vi "simple_test.vi"(8 "error in (no error)":errorcluster) -> ()   [LabVIEW 2020]
uses:
  Doc/Doc.lvclass
  Table/Table.lvclass
  Item/Item.lvclass
  Value/Value.lvclass
panel:
  out "integer_value":i64
  out "toml_string":string
  out "tables":string[](array[string])
  out "error out":errorcluster
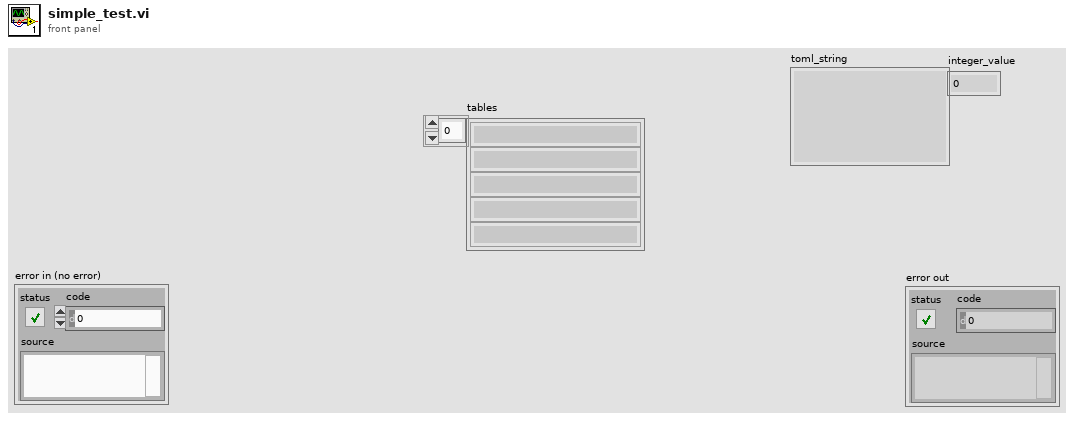
[diagram p1: front panel]
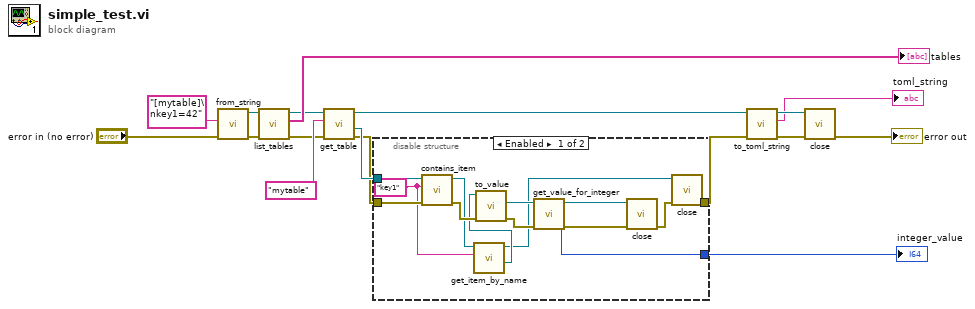
[diagram p0: block diagram]
diagram:
  n1 = call "from_string.vi"("error in (no error)"="error in (no error)", "toml"="[mytable]\nkey1=42") -> ("error out"=w14:errorcluster, "Doc out"=w15:refnum<class "Doc.lvclass">)  [unwired: 8 in]
  n2 = call "list_tables.vi"("error in (no error)"=w14, "Doc in"=w15) -> ("error out"=w5:errorcluster, "table_names"=→"tables":string[], "Doc out"=w8:refnum<class "Doc.lvclass">)  [unwired: 7 in]
  n3 = call "get_table.vi"("error in (no error)"=w5, "table_name"="mytable", "Doc in"=w8) -> ("error out"=w3:errorcluster, "Table"=w4:refnum<class "Table.lvclass">, "Doc out"=w6:refnum<class "Doc.lvclass">)  [unwired: 6 in]
  n4 = disable-structure shown="Enabled" {
    disable-tunnel: w4 -> [w31 _]
    disable-tunnel: w3 -> [w30 _]
    disable-tunnel: [w26 _] -> w2
    disable-tunnel: [w22 _] -> w1
    frame Enabled {
      w21 = "key1" ("item_name")
      n5 = call "contains_item.vi"("error in (no error)"=w30, "item_name"=w21, "Table in"=w31) -> ("error out"=w28:errorcluster, "Table out"=w19:refnum<class "Table.lvclass">)  [unwired: 6 in, 1 out]
      n6 = call "get_item_by_name.vi"("item_name"=w21, "Table in"=w19) -> ("Item"=w20:refnum<class "Item.lvclass">, "Table out"=w18:refnum<class "Table.lvclass">)  [unwired: 7 in, 1 out]
      n7 = call "to_value.vi"("error in (no error)"=w28, "Item in"=w20) -> ("error out"=w27:errorcluster, "Value out"=w29:refnum<class "Value.lvclass">)  [unwired: 8 in]
      n8 = call "get_value_for_integer.vi"("error in (no error)"=w27, "Value in"=w29) -> ("error out"=w24:errorcluster, "integer_value"=w26:i64, "Value out"=w25:refnum<class "Value.lvclass">)  [unwired: 7 in]
      n9 = call "close.vi"("error in (no error)"=w24, "Value in"=w25) -> ("error out"=w23:errorcluster)  [unwired: 9 in]
      n10 = call "close.vi"("error in (no error)"=w23, "Table in"=w18) -> ("error out"=w22:errorcluster)  [unwired: 9 in]
    }
    frame Disabled {
    }
  }
  "integer_value" <- w2
  n11 = call "to_toml_string.vi"("error in (no error)"=w1, "Doc in"=w6) -> ("error out"=w12:errorcluster, "toml_string"=→"toml_string":string, "Doc out"=w11:refnum<class "Doc.lvclass">)  [unwired: 7 in]
  n12 = call "close.vi"("error in (no error)"=w12, "Doc in"=w11) -> ("error out"=→"error out":errorcluster)  [unwired: 9 in]
